vi "webSocketVars.vi"() -> ()   [LabVIEW 2024]
uses:
  <vilib>/MediaMongrels Ltd/WebSockets/WebSockets/WebSocket Server/WebSocket Server.lvclass
  Control/webSocket_globalVar_states.ctl
panel:
  in  "webSocketStatesArray":T1[](array[typedef])
  in  "webSocketConnectionArray":refnum<class "WebSocket Server.lvclass">[](array[class])
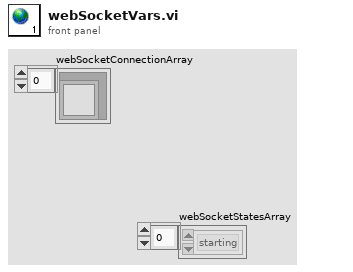
[diagram p1: front panel]
types:
  T1 = typedef "webSocket_globalVar_states.ctl" = enum16{"starting", "streaming", "close"}
diagram:
